vi "RT_WR_ADC_W_DAC.vi"() -> ()   [LabVIEW 2018]
uses:
  <vilib>/Platform/TimedLoop/XDataNode/timing_clust.ctl
  <vilib>/Platform/TimedLoop/XDataNode/nitl_modes.ctl
  <vilib>/Platform/TimedLoop/XDataNode/wakeup.ctl
  <vilib>/FPGAPlugInAG/myRIO-1900/niLvFpga_Open_myRIO-1900.vi
  <vilib>/rvi/interface/common/dynamic/niFpgaDynamicAddResources.vi
  <vilib>/Utility/error.llb/Error Cluster From Error Code.vi
  <vilib>/rvi/errors/niLvFpgaAdjustHostInterfaceError.vi
  <vilib>/FPGAPlugInAG/Dynamic/niLvFpga_Close_Dynamic.vi
  <vilib>/rvi/interface/nirviOpenFPGA/nirviOpenFPGA.xnode
  FPGA Bitfiles/ASPE2019amplifie_FPGATarget_fpgaW&RADCWDACsW_Hs6w9LSxjbU.lvbitx
  <vilib>/Platform/TimedLoop/XDataNode/XDataNode.xnode
  <vilib>/rvi/interface/nirviReadWriteControl/nirviReadWriteControl.xnode
  <vilib>/rvi/interface/nirviCloseFPGA/nirviCloseFPGA.xnode
  <vilib>/Platform/TimedLoop/XDataNode/XDNodeRunTimeDep.lvlib
  NiFpgaLv.dll
  <vilib>/rvi/interface/Simulation/niFpgaSimulationCallBeginRW.vi
panel:
  in  "DAC 3":dbl
  in  "DAC 2":dbl
  in  "DAC 1":dbl
  in  "Stop Button":bool
  in  "CH1":bool[](array[boolean])=[FALSE, FALSE, FALSE, FALSE, FALSE, TRUE, FALSE, FALSE, FALSE, FALSE, FALSE, FALSE, FALSE, FALSE, FALSE, FALSE]
  in  "CH4":bool[](array[boolean])=[FALSE, FALSE, TRUE, TRUE, FALSE, TRUE, FALSE, FALSE, FALSE, FALSE, FALSE, FALSE, FALSE, FALSE, FALSE, FALSE]
  in  "CH3":bool[](array[boolean])=[FALSE, FALSE, TRUE, FALSE, FALSE, TRUE, FALSE, FALSE, FALSE, FALSE, FALSE, FALSE, FALSE, FALSE, FALSE, FALSE]
  in  "CH2":bool[](array[boolean])=[FALSE, FALSE, FALSE, TRUE, FALSE, TRUE, FALSE, FALSE, FALSE, FALSE, FALSE, FALSE, FALSE, FALSE, FALSE, FALSE]
  out "ADC 4":dbl(graph)=-2.0281672948105642
  out "ADC 3":dbl(graph)=-0.5364908372369804
  out "ADC 2":dbl(graph)=-0.0015258556235409
  out "ADC 1":dbl(graph)=-0.0015258556235409
  in  "us":u32=150
  out "Finished Late? [i-1]":bool
  # "Enter the desired voltage you want to input to the current amplifier connected to voice coil. \n10 V corresponds to 1 A to coil"
  # "You can read the voltage ouput of sensors in the following plots"
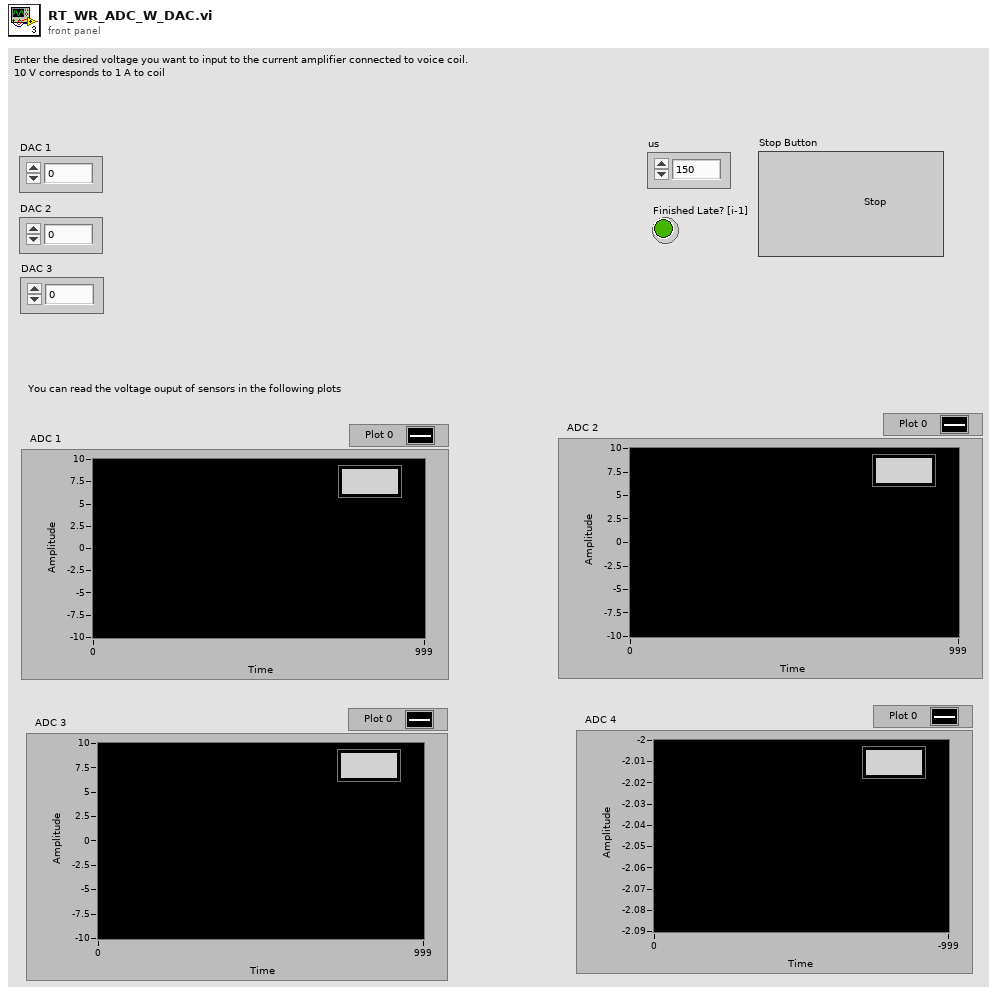
[diagram p1: front panel]
types:
  T1 = typedef "XDNodeRunTimeDep.lvlib/timing_clust.ctl" = cluster{"Expected End [f-1]":u64, "Actual End [f-1]":u64, "Finished Late? [f-1]":bool, "Expected End [i-1]":u64, "Actual End [i-1]":u64, "Finished Late? [i-1]":bool, "Expected Start [i]":u64, "Actual Start [i]":u64, "Expected Start [f]":u64, "Actual Start [f]":u64, "Source Name":string, "Structure Name":string, "Period":i64, "Deadline":i64, "Offset":i64, "Start":i64, "Priority":i32, "Timeout":i32, "Mode":T2, "Wakeup Reason":T3, "Error":errorcluster, "Source Type":string, "Secondary Source Type":string, "Global End Time":u64, "Global Start Time":u64, "Frame Duration":u64, "Iteration Duration":u64, "Assigned CPU":i32, "I/O Scan Engine Mode":u32}
  T2 = typedef "XDNodeRunTimeDep.lvlib/nitl_modes.ctl" = enum32{"No Change", "Process missed periods, maintain original phase", "Discard missed periods, maintain original phase", "Process missed periods, ignore original phase", "Discard missed periods, ignore original phase"}
  T3 = typedef "XDNodeRunTimeDep.lvlib/wakeup.ctl" = enum32{"Normal", "Aborted", "Asynchronous wakeup", "Timing source error", "Timed loop error", "Timeout"}
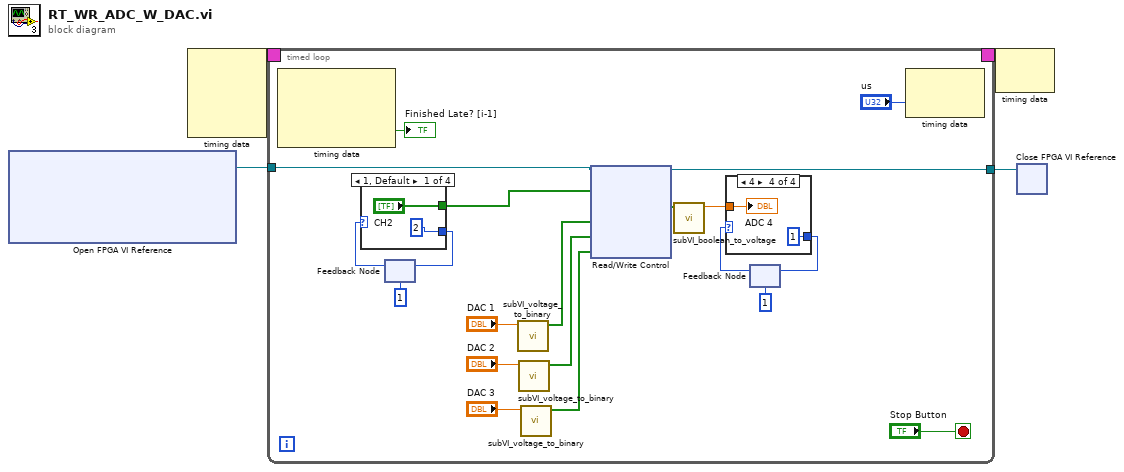
[diagram p0: block diagram]
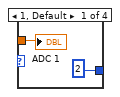
[diagram p2: hidden frame]
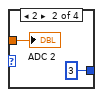
[diagram p3: hidden frame]
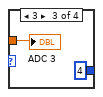
[diagram p4: hidden frame]
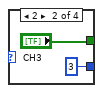
[diagram p5: hidden frame]
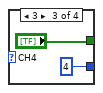
[diagram p6: hidden frame]
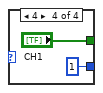
[diagram p7: hidden frame]
diagram:
  n1 = xnode "Open FPGA VI Reference"() -> ("FPGA VI Reference Out"=w2:refnum<k20>)  [unwired: 2 in, 1 out]
  n2 = node-c288() -> (w4:T1)  [unwired: 4 in]
  n3 = timed-loop {
    tunnel: w2 -> [w24]
    timing: w4 -> [_]
    timing-out: [_] -> w3
    tunnel: [w5] -> w1
    stop <- "Stop Button" stop-if-true
    n4 = node-c288() -> (→"Finished Late? [i-1]":bool)  [unwired: 1 in, 3 out]
    n5 = feedback #1(1) -> (w22:i32)
    n6 = case shown="1, Default" w22 {
      tunnel: ["CH2" "CH3" "CH4" "CH1"] -> w19
      tunnel: [2 3 4 1] -> w20
      frame 1, Default {
      }
      frame 2 {
      }
      frame 3 {
      }
      frame 4 {
      }
    }
    n7 = feedback-in #1(w20) -> ()
    n8 = call "subVI_voltage_to_binary.vi"("voltage"="DAC 1") -> ("binary"=w11:bool[])  [unwired: 10 in]
    n9 = call "subVI_voltage_to_binary.vi"("voltage"="DAC 2") -> ("binary"=w10:bool[])  [unwired: 10 in]
    n10 = call "subVI_voltage_to_binary.vi"("voltage"="DAC 3") -> ("binary"=w9:bool[])  [unwired: 10 in]
    n11 = xnode "Read/Write Control"("FPGA VI Reference In"=w24, "ADC write"=w19, "DAC 1 write"=w11, "DAC 2 write"=w10, "DAC 3 write"=w9) -> ("FPGA VI Reference Out"=w5:refnum<k20>, "ADC read"=w12:bool[])  [unwired: 1 in, 1 out]
    n12 = call "subVI_boolean_to_voltage.vi"("ADC read"=w12) -> ("V"=w15:dbl)  [unwired: 10 in]
    n13 = feedback #2(1) -> (w18:i32)
    n14 = case shown="4" w18 {
      tunnel: [2 3 4 1] -> w16
      tunnel: w15 -> [w30 w32 w34 w36]
      frame 1, Default {
        "ADC 1" <- w30
      }
      frame 2 {
        "ADC 2" <- w32
      }
      frame 3 {
        "ADC 3" <- w34
      }
      frame 4 {
        "ADC 4" <- w36
      }
    }
    n15 = feedback-in #2(w16) -> ()
    n16 = node-c288("us") -> ()  [unwired: 1 in, 1 out]
  }
  n17 = node-c288(w3) -> ()  [unwired: 1 out]
  n18 = xnode "Close FPGA VI Reference"("FPGA VI Reference In"=w1) -> ()  [unwired: 1 in, 1 out]
